vi "DQMH-GenNet Add Notifier To Variant.vi"(10 "Wait Notifier":refnum<notifier>, 11 "Event Data IN":variant) -> (3 "Variant OUT":variant)   [LabVIEW 2022 SP3, in "hse-gennet.lvlib"]
doc: "HSE: If a notifier reference is given, stores it as an attribute inside the Message Data variant. The notification data type is variant.\n\n____\nHAMPEL SOFTWARE ENGINEERING v3.8.0 (2023-12-18 14:41)"
uses:
  hse-gennet.lvlib
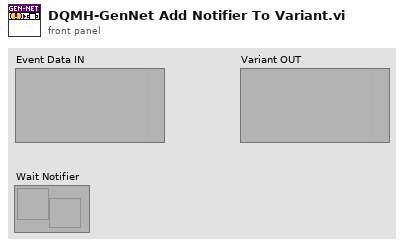
[diagram p1: front panel]
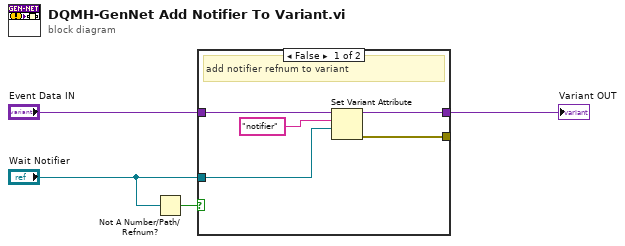
[diagram p0: block diagram]
diagram:
  n1 = Not A Number/Path/Refnum?(number/path/refnum="Wait Notifier") -> (NaN/Path/Refnum?=w2:bool)
  n2 = case shown="False" w2 {
    tunnel: [w6 w10] -> w4
    tunnel: "Event Data IN" -> [w8 w10]
    tunnel: "Wait Notifier" -> [w7 _]
    tunnel: [w5 _] -> _
    frame False {
      # "add notifier refnum to variant"
      n3 = Set Variant Attribute(Variant=w8, name="notifier", value=w7) -> (Variant out=w6:variant, error out=w5:errorcluster)  [unwired: 1 in, 1 out]
    }
    frame True {
      # "invalid notifier refnum: do nothing"
    }
  }
  "Variant OUT" <- w4
